vi "Set DAC (Raw).vi"(7 "Channel Select":T1, 8 "error in (no error)":errorcluster, 10 "DAC Value (Raw)":u16, 11 "DAC8552 in":refnum<class "LINX-DAC8552.lvclass">) -> (0 "error out":errorcluster, 3 "DAC8552 out":refnum<class "LINX-DAC8552.lvclass">)   [LabVIEW 2020, in "LINX-DAC8552.lvclass"]
doc: "Sets the raw DAC output level for the specified channel(s)."
uses:
  LINX-DAC8552.lvclass
  Channel Select.ctl
  Power Down Mode.ctl
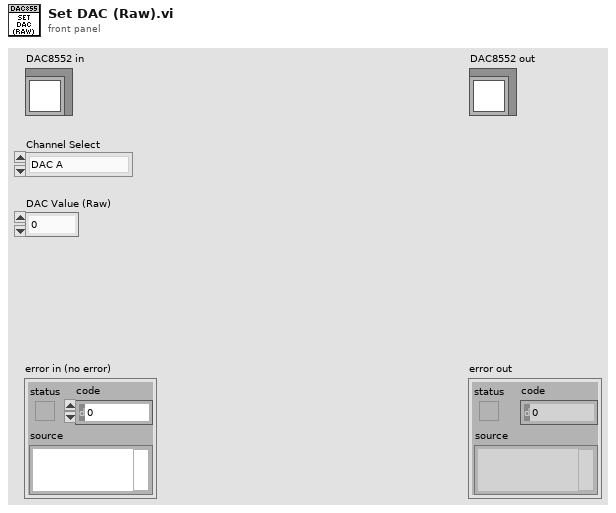
[diagram p1: front panel]
types:
  T1 = typedef "LINX-DAC8552.lvclass/Channel Select.ctl" = enum8{"DAC A", "DAC B", "Both"}
  T2 = typedef "LINX-DAC8552.lvclass/Power Down Mode.ctl" = enum8{"On - Normal Operation", "Off - 1kOhm", "Off - 100kOhm", "Off - High Impedence"}
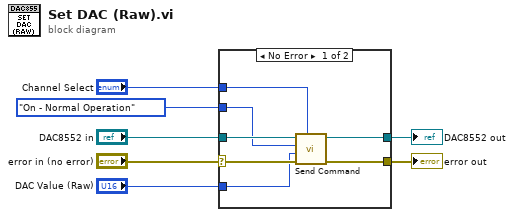
[diagram p0: block diagram]
diagram:
  n1 = case shown="No Error" "error in (no error)" {
    selector: "error in (no error)" -> [w12 w16]
    tunnel: [w11 w16] -> w6
    tunnel: [w13 w15] -> w4
    tunnel: "DAC8552 in" -> [w14 w15]
    tunnel: Power_Down_Mode."On - Normal Operation" ("Power Down Mode") -> [w10 _]
    tunnel: "Channel Select" -> [w9 _]
    tunnel: "DAC Value (Raw)" -> [w8 _]
    frame No Error {
      n2 = call "Send Command.vi"("Channel Select"=w9, "error in (no error)"=w12, "Data"=w8, "Power Down Mode"=w10, "LINX-DAC8552 in"=w14) -> ("error out"=w11:errorcluster, "LINX-DAC8552 out"=w13:refnum<class "LINX-DAC8552.lvclass">)  [unwired: 5 in]
    }
    frame Error {
    }
  }
  "error out" <- w6
  "DAC8552 out" <- w4
